vi "Plot Closed.vi"(8 "error in (no error)":errorcluster, 10 "Closed plot":refnum<class "Message Enqueuer.lvclass">, 11 "Application Controller in":refnum<class "Application Controller.lvclass">) -> (0 "error out":errorcluster, 3 "Application Controller out":refnum<class "Application Controller.lvclass">)   [LabVIEW 2018, in "Application Controller.lvclass"]
uses:
  Application Controller.lvclass
  <vilib>/ActorFramework/Message Enqueuer/Message Enqueuer.lvclass
  Application Controller.lvclass/Application Controller.ctl
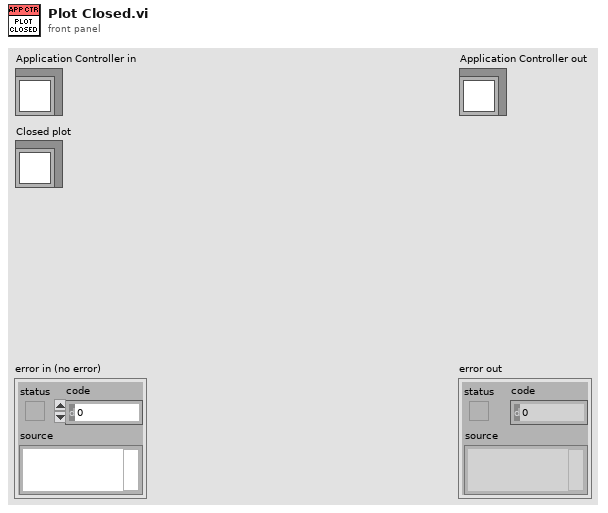
[diagram p1: front panel]
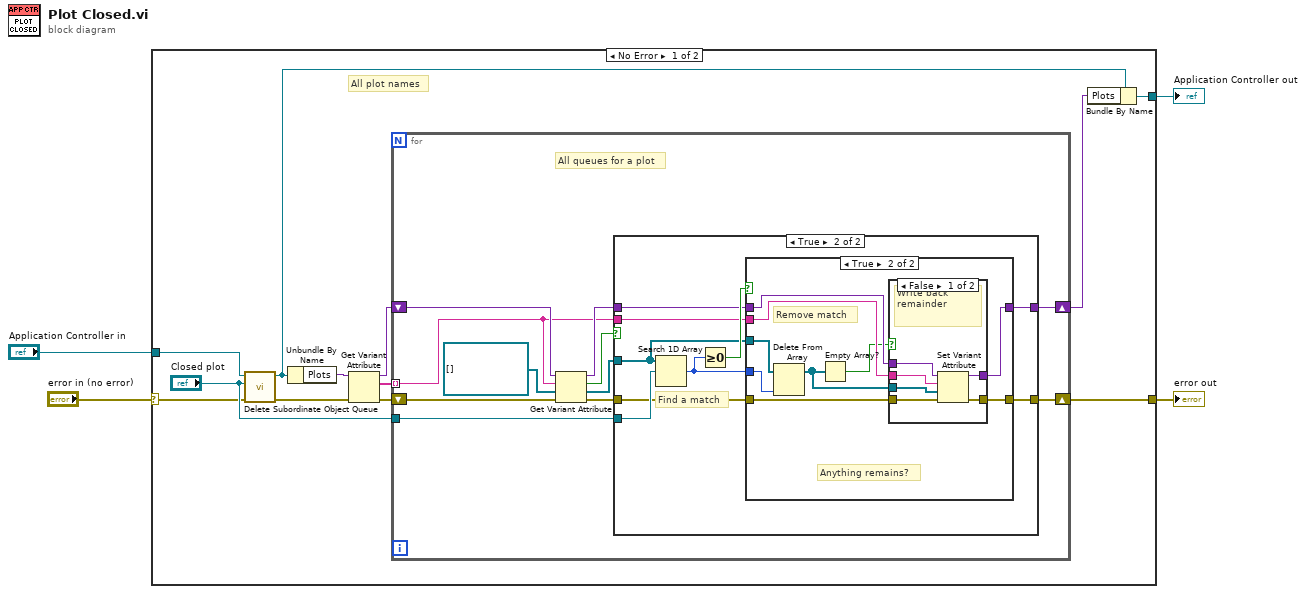
[diagram p0: block diagram]
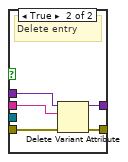
[diagram p4: hidden frame]
diagram:
  n1 = case shown="No Error" "error in (no error)" {
    selector: "error in (no error)" -> [w9 w62]
    tunnel: [w5 w62] -> w3
    tunnel: [w10 w61] -> w1
    tunnel: "Application Controller in" -> [w7 w61]
    frame No Error {
      # "All plot names"
      n2 = call-dynamic "Delete Subordinate Object Queue.vi"("error in (no error)"=w9, "Caller-To-Actor Enqueuer"="Closed plot", "Template Module in"=w7) -> ("error out"=w8:errorcluster, "Template Module out"=w6:refnum<class "Application Controller.lvclass">)  [unwired: 7 in]
      n3 = Unbundle By Name(w6) -> ("Plots"=w16:variant)
      n4 = Get Variant Attribute(Variant=w16, error in=w8) -> (duplicate Variant=w14:variant, names=w15:string[], error out=w13:errorcluster)  [unwired: 2 in, 1 out]
      n5 = for {
        tunnel: w15 -> [w20] mode=indexing
        shift-right: [w18] -> w5
        shift-left: w13 -> [w26]
        tunnel: "Closed plot" -> [w23]
        shift-right: [w17] -> w12
        shift-left: w14 -> [w27]
        # "All queues for a plot"
        n6 = Get Variant Attribute(Variant=w27, name=w20, default value (empty Variant)=refnum<class "Message Enqueuer.lvclass">[] [] ("Plot enqueuers"), error in=w26) -> (duplicate Variant=w21:variant, found=w22:bool, value=w24:refnum<class "Message Enqueuer.lvclass">[], error out=w19:errorcluster)
        n7 = case shown="True" w22 {
          tunnel: w24 -> [_ w36]
          tunnel: w23 -> [_ w35]
          tunnel: w21 -> [w28 w34]
          tunnel: w20 -> [_ w33]
          tunnel: w19 -> [w29 w32]
          tunnel: [w29 w31] -> w18
          tunnel: [w28 w30] -> w17
          frame False {
          }
          frame True {
            # "Find a match"
            n8 = Search 1D Array(1D array=w36, element=w35) -> (index of element=w37:i32)  [unwired: 1 in]
            n9 = Greater Or Equal To 0?(x=w37) -> (x >= 0?=w38:bool)
            n10 = case shown="True" w38 {
              tunnel: w36 -> [_ w49]
              tunnel: w37 -> [_ w48]
              tunnel: w34 -> [w40 w46]
              tunnel: [w40 w47] -> w30
              tunnel: w33 -> [_ w45]
              tunnel: w32 -> [w39 w44]
              tunnel: [w39 w43] -> w31
              frame False {
              }
              frame True {
                # "Anything remains?"
                # "Remove match"
                n11 = Delete From Array(array=w49, index=w48) -> (array with subset deleted=w42:refnum<class "Message Enqueuer.lvclass">[])  [unwired: 1 in, 1 out]
                n12 = Empty Array?(array=w42) -> (empty?=w41:bool)
                n13 = case shown="False" w41 {
                  tunnel: [w55 w58] -> w47
                  tunnel: w46 -> [w54 w57]
                  tunnel: w45 -> [w53 w56]
                  tunnel: w44 -> [w52 w60]
                  tunnel: [w51 w59] -> w43
                  tunnel: w42 -> [w50 _]
                  frame False {
                    # "Write back \nremainder"
                    n14 = Set Variant Attribute(Variant=w54, name=w53, value=w50, error in=w52) -> (Variant out=w55:variant, error out=w51:errorcluster)  [unwired: 1 out]
                  }
                  frame True {
                    # "Delete entry"
                    n15 = Delete Variant Attribute(4:w60, 6:w56, 7:w57) -> (0:w59:errorcluster, 3:w58:variant)  [unwired: 1 out]
                  }
                }
              }
            }
          }
        }
      }
      n16 = Bundle By Name(cluster=w6, "Plots"=w12) -> (w10:refnum<class "Application Controller.lvclass">)
    }
    frame Error {
    }
  }
  "error out" <- w3
  "Application Controller out" <- w1
